vi "scan2d_close_log.vi"(8 "error in (no error)":errorcluster, 11 "scan_2d in":refnum<class "scan_2d.lvclass">) -> (0 "error out":errorcluster, 3 "scan_2d out":refnum<class "scan_2d.lvclass">)   [LabVIEW 2015, in "scan_2d.lvclass"]
uses:
  scan_2d.lvclass
  scan_2d.lvclass/scan_2d.ctl
  scan_2d_hdf5_log/scan_2d_hdf5_log.lvclass
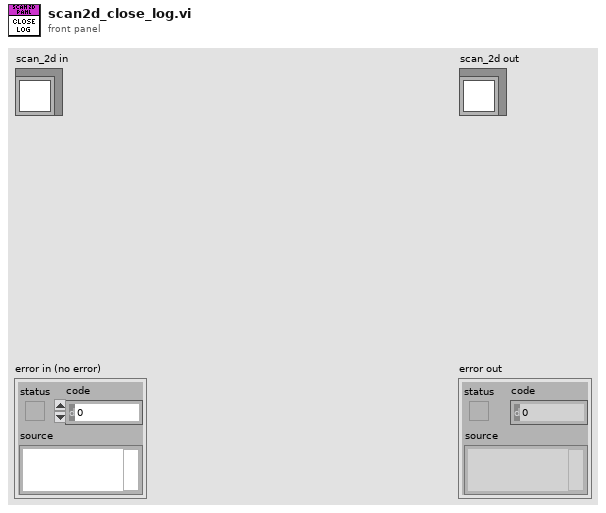
[diagram p1: front panel]
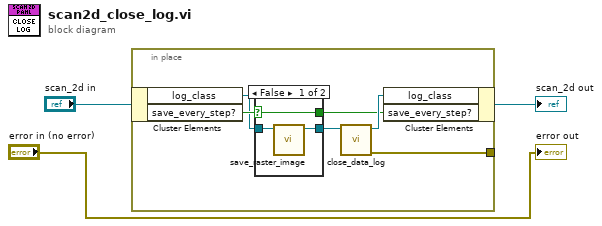
[diagram p0: block diagram]
diagram:
  n1 = in-place {
    in-place-border: [w6] -> _
    n2 = in-place-cluster #1("scan_2d in") -> ("log_class"=w8:refnum<class "scan_2d_hdf5_log.lvclass">, "save_every_step?"=w9:bool)
    n3 = case shown="False" w9 {
      selector: w9 -> [w10 w14]
      tunnel: w8 -> [w12 w13]
      tunnel: [w11 w13] -> w7
      tunnel: [w10 w14] -> w4
      frame False {
        n4 = call "save_raster_image.vi"("scan_2d_hdf5_log in"=w12) -> ("scan_2d_hdf5_log out"=w11:refnum<class "scan_2d_hdf5_log.lvclass">)  [unwired: 9 in, 1 out]
      }
      frame True {
      }
    }
    n5 = call-dynamic "close_data_log.vi"("scan_hdf5_log in"=w7) -> ("error out"=w6:errorcluster, "scan_hdf5_log out"=w5:refnum<class "scan_2d_hdf5_log.lvclass">)  [unwired: 9 in]
    n6 = in-place-cluster #1("log_class"=w5, "save_every_step?"=w4) -> (→"scan_2d out":refnum<class "scan_2d.lvclass">)
  }
  "error out" <- "error in (no error)"
